vi "Script Error VI.vi"(4 "Error Code":i32, 6 "Error Name":string, 7 "Error Arguments Window Ref":refnum<vi>, 8 "error in":errorcluster, 9 "Error Description":string, 10 "Library Path":path, 11 "VI Ref Error in":refnum<vi>) -> (0 "error out":errorcluster, 3 "Custom Error VI Ref":refnum<vi>)   [LabVIEW 2020, in "ConstantErrorsMaker.lvlib"]
uses:
  ConstantErrorsMaker.lvlib
  <vilib>/Utility/traverseref.llb/TRef TravTarget.ctl
  <vilib>/Utility/miscctls.llb/LVPositionTypeDef.ctl
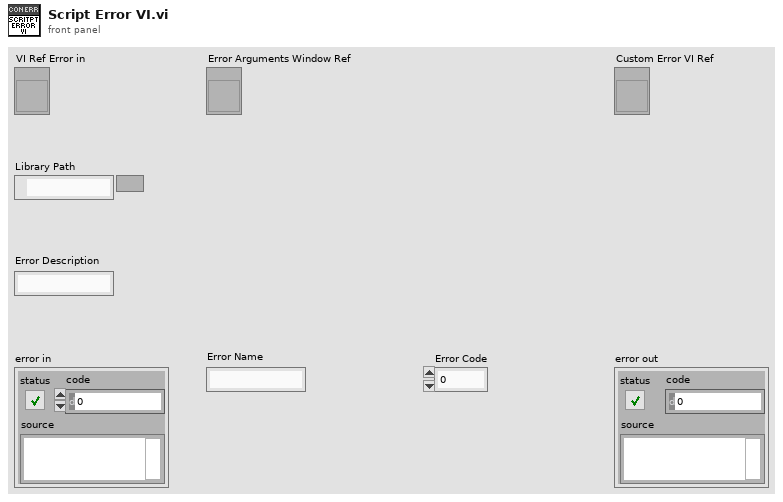
[diagram p1: front panel]
types:
  T1 = typedef "TRef TravTarget.ctl" = enum16{"FP", "BD", "Other"}
  T2 = typedef "LVPositionTypeDef.ctl" = cluster{"Left":i32, "Top":i32}
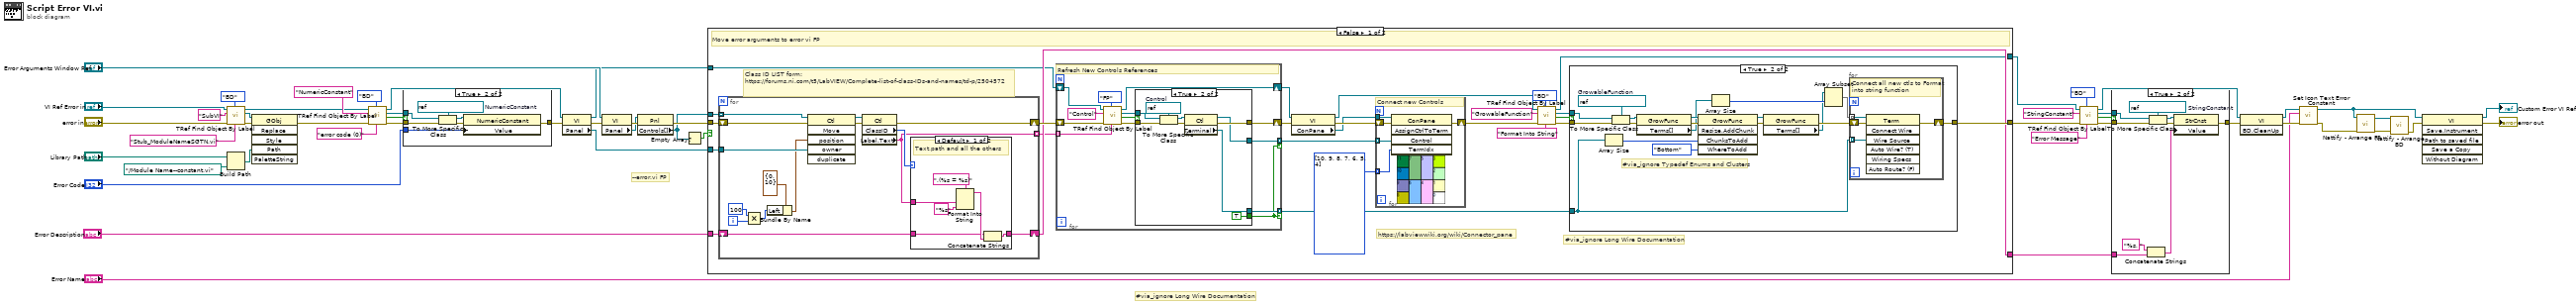
[diagram p0: block diagram]
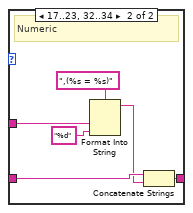
[diagram p4: hidden frame]
diagram:
  # "#via_ignore Long Wire Documentation"
  # "--error.vi FP"
  n1 = call <vilib>:"TRef Find Object By Label.vi"("Label"="Stub_ModuleNameSGTN.vi", "Traverse Target"=TRef_TravTarget."BD", "error in (no error)"="error in", "Class Name"="SubVI", "VI Ref"="VI Ref Error in") -> ("error out"=w52:errorcluster, "Found Obj Ref"=w31:refnum<vi>, "dup VI Ref"=w26:refnum<vi>)  [unwired: 3 in, 1 out]
  n2 = Build Path(base path="Library Path", name or relative path=path "../Module Name--constant.vi") -> (appended path=w34:path)
  n3 = invoke class="GObj" method="Replace"(reference=w31, error in=w52, "Path"=w34) -> (error out=w50:errorcluster)  [unwired: 3 in, 5 out]
  n4 = call <vilib>:"TRef Find Object By Label.vi"("Label"="error code (0)", "Traverse Target"=TRef_TravTarget."BD", "error in (no error)"=w50, "Class Name"="NumericConstant", "VI Ref"=w26) -> ("error out"=w49:errorcluster, "Found?"=w25:bool, "Found Obj Ref"=w24:refnum<vi>, "dup VI Ref"=w13:refnum<vi>)  [unwired: 3 in]
  n5 = case shown="True" w25 {
    tunnel: w49 -> [w53 w60]
    tunnel: w24 -> [_ w57]
    tunnel: "Error Code" -> [_ w54]
    tunnel: [w53 w58] -> w44
    frame False {
    }
    frame True {
      w56 = refnum<vi> refnum  # NumericConstant
      n6 = To More Specific Class(target class=w56, reference=w57, error in=w60) -> (specific class reference=w55:refnum<vi>, error out=w59:errorcluster)
      n7 = property class="NumericConstant"(reference=w55, error in=w59, "Value"=w54) -> (error out=w58:errorcluster)  [unwired: 1 out]
    }
  }
  n8 = property class="VI"(reference=w13, error in=w44) -> (reference out=w11:refnum<vi>, error out=w45:errorcluster, "Panel"=w14:refnum<vi>)
  n9 = property class="VI"(reference="Error Arguments Window Ref", error in=w45) -> (error out=w47:errorcluster, "Panel"=w17:refnum<vi>)  [unwired: 1 out]
  n10 = property class="Pnl"(reference=w17, error in=w47) -> (error out=w46:errorcluster, "Controls[]"=w15:refnum<vi>[])  [unwired: 1 out]
  n11 = Empty Array?(array=w15) -> (empty?=w16:bool)
  n12 = case shown="False" w16 {
    tunnel: w46 -> [w85 w166]
    tunnel: w15 -> [w69 _]
    tunnel: w14 -> [w78 _]
    tunnel: [w83 w166] -> w43
    tunnel: "Error Description" -> [w77 w165]
    tunnel: [w76 w165] -> w7
    tunnel: w11 -> [w66 w164]
    tunnel: [w75 w164] -> w10
    frame False {
      # "#via_ignore Long Wire Documentation"
      # "https://labviewwiki.org/wiki/Connector_pane"
      # "Class ID LIST form:\nhttps://forums.ni.com/t5/LabVIEW/Complete-list-of-class-IDs-and-names/td-p/2504572"
      # "Move error arguments to error vi FP"
      n13 = for {
        tunnel: w69 -> [w143] mode=indexing
        tunnel: w78 -> [w142]
        shift-right: [w144] -> w82
        shift-left: w85 -> [w146]
        shift-right: [w137] -> w76
        shift-left: w77 -> [w138]
        tunnel: [w136] -> w68 mode=indexing
        i -> [w134]
        n14 = Multiply(x=100, y=w134) -> (x*y=w133:i32)
        n15 = Bundle By Name(cluster=T2 {"Left"=0, "Top"=10} ("position"), "Left"=w133) -> (w135:T2)
        n16 = invoke class="Ctl" method="Move"(reference=w143, error in=w146, "position"=w135, "owner"=w142) -> (reference out=w140:refnum<vi>, error out=w145:errorcluster)  [unwired: 2 in, 4 out]
        n17 = property class="Ctl"(reference=w140, error in=w145) -> (error out=w144:errorcluster, "ClassID"=w139:u32, "Label.Text"=w136:string)  [unwired: 1 out]
        n18 = case shown="Default" w139 {
          tunnel: w138 -> [w148 w158]
          tunnel: [w149 w157] -> w137
          tunnel: w136 -> [w147 w156]
          frame Default {
            # "Text,path and all the others"
            n19 = Format Into String(format string=",(%s = %s)", w147, "%s" ("string")) -> (resulting string=w150:string)  [unwired: 2 in, 1 out]
            n20 = Concatenate Strings(w148, w150) -> (w149:string)
          }
          frame 17..23, 32..34 {
            # "Numeric"
            n21 = Format Into String(format string=",(%s = %s)", w156, "%d" ("string")) -> (resulting string=w153:string)  [unwired: 2 in, 1 out]
            n22 = Concatenate Strings(w158, w153) -> (w157:string)
          }
        }
      }
      n23 = for {
        tunnel: w68 -> [w118] mode=indexing
        shift-right: [w119] -> w81
        shift-left: w82 -> [w121]
        tunnel: [w114] -> w67 mode=indexing if=w109
        shift-right: [w111] -> w65
        shift-left: w66 -> [w113]
        tunnel: [w110] -> w62 mode=indexing if=w109
        # "Refresh New Controls References"
        n24 = call <vilib>:"TRef Find Object By Label.vi"("Label"=w118, "Traverse Target"=TRef_TravTarget."FP", "error in (no error)"=w121, "Class Name"="Control", "VI Ref"=w113) -> ("error out"=w120:errorcluster, "Found?"=w112:bool, "Found Obj Ref"=w116:refnum<vi>, "dup VI Ref"=w111:refnum<vi>)  [unwired: 3 in]
        n25 = case shown="True" w112 {
          tunnel: w116 -> [_ w128]
          tunnel: [_ w125] -> w114
          tunnel: w120 -> [w122 w131]
          tunnel: [w122 w129] -> w119
          tunnel: [_ TRUE] -> w109
          tunnel: [_ w123] -> w110
          frame False {
          }
          frame True {
            w126 = refnum<vi> refnum  # Control
            n26 = To More Specific Class(target class=w126, reference=w128, error in=w131) -> (specific class reference=w127:refnum<vi>, error out=w130:errorcluster)
            n27 = property class="Ctl"(reference=w127, error in=w130) -> (reference out=w123:refnum<vi>, error out=w129:errorcluster, "Terminal"=w125:refnum<vi>)
          }
        }
      }
      n28 = property class="VI"(reference=w65, error in=w81) -> (reference out=w64:refnum<vi>, error out=w80:errorcluster, "ConPane"=w63:refnum<vi>)
      n29 = for {
        tunnel: w63 -> [w161]
        shift-right: [w162] -> w79
        shift-left: w80 -> [w163]
        tunnel: w62 -> [w160] mode=indexing
        tunnel: i32[] [10, 9, 8, 7, 6, 5, 4] -> [w159] mode=indexing
        # "Connect new Controls"
        n30 = invoke class="ConPane" method="AssignCtrlToTerm"(reference=w161, error in=w163, "Control"=w160, "TermIdx"=w159) -> (error out=w162:errorcluster)  [unwired: 1 in, 4 out]
      }
      n31 = call <vilib>:"TRef Find Object By Label.vi"("Label"="Format Into String", "Traverse Target"=TRef_TravTarget."BD", "error in (no error)"=w79, "Class Name"="GrowableFunction", "VI Ref"=w64) -> ("error out"=w84:errorcluster, "Found?"=w72:bool, "Found Obj Ref"=w71:refnum<vi>, "dup VI Ref"=w75:refnum<vi>)  [unwired: 3 in]
      n32 = case shown="True" w72 {
        tunnel: w84 -> [w86 w104]
        tunnel: w71 -> [_ w98]
        tunnel: [w86 w99] -> w83
        tunnel: w67 -> [_ w87]
        frame False {
        }
        frame True {
          w97 = refnum<vi> refnum  # GrowableFunction
          # "#via_ignore Typedef Enums and Clusters"
          n33 = Array Size(array=w87) -> (size(s)=w95:i32)
          n34 = To More Specific Class(target class=w97, reference=w98, error in=w104) -> (specific class reference=w93:refnum<vi>, error out=w103:errorcluster)
          n35 = property class="GrowFunc"(reference=w93, error in=w103) -> (reference out=w92:refnum<vi>, error out=w101:errorcluster, "Terms[]"=w91:refnum<vi>[])
          n36 = invoke class="GrowFunc" method="Resize.AddChunk"(reference=w92, error in=w101, "ChunksToAdd"=w95, "WhereToAdd"=enum8{"Bottom", "Top"}."Bottom" ("Where To Add")) -> (reference out=w94:refnum<vi>, error out=w102:errorcluster)  [unwired: 1 in, 3 out]
          n37 = Array Size(array=w91) -> (size(s)=w90:i32)
          n38 = property class="GrowFunc"(reference=w94, error in=w102) -> (error out=w100:errorcluster, "Terms[]"=w89:refnum<vi>[])  [unwired: 1 out]
          n39 = Array Subset(array=w89, index=w90) -> (w88:refnum<vi>[])  [unwired: 1 in]
          n40 = for {
            tunnel: w88 -> [w106] mode=indexing
            tunnel: w87 -> [w105] mode=indexing
            shift-right: [w107] -> w99
            shift-left: w100 -> [w108]
            # "Connect all new ctls to Format into string function"
            n41 = invoke class="Term" method="Connect Wire"(reference=w106, error in=w108, "Wire Source"=w105) -> (error out=w107:errorcluster)  [unwired: 4 in, 6 out]
          }
        }
      }
    }
    frame True {
      # "No Error Arguments"
    }
  }
  n42 = call <vilib>:"TRef Find Object By Label.vi"("Label"="Error Message", "Traverse Target"=TRef_TravTarget."BD", "error in (no error)"=w43, "Class Name"="StringConstant", "VI Ref"=w10) -> ("error out"=w48:errorcluster, "Found?"=w20:bool, "Found Obj Ref"=w19:refnum<vi>, "dup VI Ref"=w12:refnum<vi>)  [unwired: 3 in]
  n43 = case shown="True" w20 {
    tunnel: w48 -> [w167 w176]
    tunnel: w19 -> [_ w173]
    tunnel: [w167 w174] -> w42
    tunnel: w7 -> [_ w170]
    frame False {
    }
    frame True {
      w172 = refnum<vi> refnum  # StringConstant
      n44 = Concatenate Strings("%s, " ("string"), w170) -> (w169:string)
      n45 = To More Specific Class(target class=w172, reference=w173, error in=w176) -> (specific class reference=w171:refnum<vi>, error out=w175:errorcluster)
      n46 = property class="StrCnst"(reference=w171, error in=w175, "Value"=w169) -> (error out=w174:errorcluster)  [unwired: 1 out]
    }
  }
  n47 = invoke class="VI" method="BD.CleanUp"(reference=w12, error in=w42) -> (reference out=w3:refnum<vi>, error out=w37:errorcluster)  [unwired: 1 in, 1 out]
  n48 = call "Set Icon Text Error Constant.vi"("error in"=w37, "Text"="Error Name", "VI in"=w3) -> ("error out"=w41:errorcluster, "VI out"=w4:refnum<vi>)  [unwired: 7 in]
  n49 = call "Nattify - Arrange FP.vi"("VI in"=w4, "error in"=w41) -> ("VI out"=w5:refnum<vi>, "error out"=w39:errorcluster)  [unwired: 12 in]
  n50 = call "Nattify - Arrange BD.vi"("VI in"=w5, "error in"=w39) -> ("error out"=w38:errorcluster)  [unwired: 13 in]
  n51 = invoke class="VI" method="Save.Instrument"(reference=w4, error in=w38) -> (reference out=→"Custom Error VI Ref":refnum<vi>, error out=→"error out":errorcluster)  [unwired: 4 in, 4 out]
